vi "list and create PG message table 64.vi"(8 "error in":errorcluster, 9 "serial_n name":string="serial_n1_seq", 10 "table name":string, 11 "conn":u64) -> (0 "error out":errorcluster, 3 "conn_out":u64)   [LabVIEW 2019, in "PostgreSQL.lvlib"]
uses:
  PostgreSQL.lvlib
  PostgreSQL2LabVIEW/libpqlv64/src/PQresultErrorMessage.vi
  PostgreSQL2LabVIEW/libpqUtility64/src/PQclear.vi
  PostgreSQL2LabVIEW/libpqlv64/src/PQsendQuery.vi
  PostgreSQL2LabVIEW/libpqlv64/src/PQgetResult.vi
  PostgreSQL2LabVIEW/libpqlv64/src/PQresultStatus.vi
  PostgreSQL2LabVIEW/libpqUtility64/src/PQgetColumn.vi
  PostgreSQL2LabVIEW/libpqlv64/src/PQclear.vi
  PostgreSQL2LabVIEW/libpqUtility64/src/PQfetchTables.vi
  PostgreSQL2LabVIEW/libpqlv64/src/PQgetvalue.vi
  PostgreSQL2LabVIEW/libpqlv64/src/PQntuples.vi
  PostgreSQL2LabVIEW/libpqUtility64/libpqutility64.lvlib
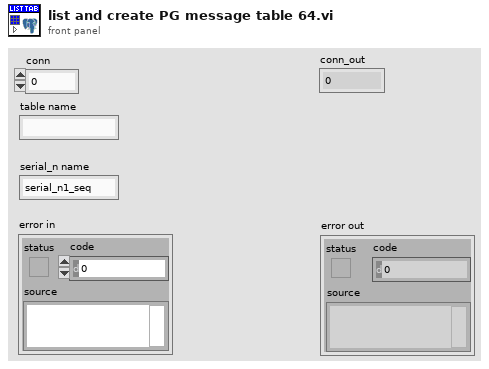
[diagram p1: front panel]
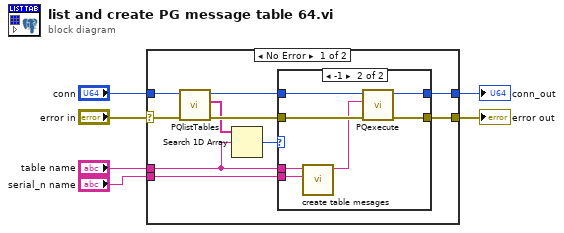
[diagram p0: block diagram]
diagram:
  n1 = case shown="No Error" "error in" {
    selector: "error in" -> [w14 w27]
    tunnel: "conn" -> [w11 w26]
    tunnel: [w16 w26] -> w4
    tunnel: [w15 w27] -> w3
    tunnel: "table name" -> [w8 _]
    tunnel: "serial_n name" -> [w10 _]
    frame No Error {
      n2 = call "PQlistTables.vi"("error in"=w14, "conn"=w11) -> ("error out"=w13:errorcluster, "Data"=w9:string[], "conn_out"=w12:u64)  [unwired: 7 in]
      n3 = Search 1D Array(1D array=w9, element=w8) -> (index of element=w7:i32)  [unwired: 1 in]
      n4 = case shown="-1" w7 {
        tunnel: w12 -> [w18 w25]
        tunnel: [w18 w23] -> w16
        tunnel: w13 -> [w17 w24]
        tunnel: [w17 w22] -> w15
        tunnel: w8 -> [_ w20]
        tunnel: w10 -> [_ w19]
        frame 0, Default {
        }
        frame -1 {
          n5 = call "create table mesages.vi"("serial_n name"=w19, "table name"=w20) -> ("create table parameters"=w21:string)  [unwired: 9 in]
          n6 = call "PQexecute.vi"("error in"=w24, "SQL querry"=w21, "conn"=w25) -> ("error out"=w22:errorcluster, "conn_out"=w23:u64)  [unwired: 7 in]
        }
      }
    }
    frame Error {
    }
  }
  "conn_out" <- w4
  "error out" <- w3
